vi "solar_voy Write (HS).vi"(4 "HDR_GUID":string, 6 "Suppress Errors? (T)":bool=TRUE, 7 "TARGET":string, 8 "error in (no error)":errorcluster, 10 "HANDSHAKE":T1, 11 "Voyager Refnum in":T2) -> (0 "error out":errorcluster, 3 "Voyager Refnum out":T2)   [LabVIEW 2018]
doc: "This writes the 'HANDSHAKE' packet used by the LINC interface."
uses:
  solar_voy_ctl Voyager Refnum.ctl
  solar_voy_def/solar_voy_def_ctl HANDSHAKE.ctl
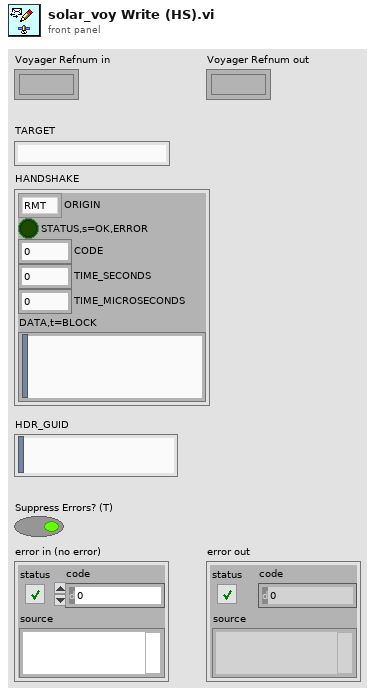
[diagram p1: front panel]
types:
  T1 = typedef "solar_voy_def_ctl HANDSHAKE.ctl" = cluster{"ORIGIN":enum8{"RMT", "LCL"}, "STATUS,s=OK,ERROR":bool, "CODE":i32, "TIME_SECONDS":u32, "TIME_MICROSECONDS":u32, "DATA,t=BLOCK":string}
  T2 = typedef "solar_voy_ctl Voyager Refnum.ctl" = refnum<k1>
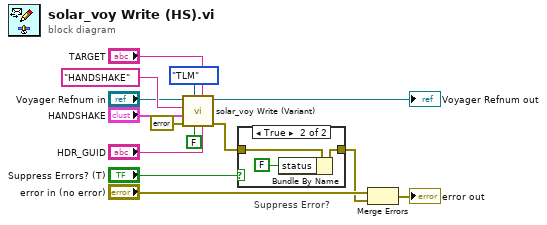
[diagram p0: block diagram]
diagram:
  n1 = call "solar_voy Write (Variant).vi"("HDR_GUID"="HDR_GUID", "TARGET"="TARGET", "Suppress Errors? (T)"=FALSE, "CMD"=enum8{"CMD", "TLM"}."TLM", "error in (no error)"=errorcluster {"status"=FALSE, "code"=0, "source"=""}, "Variant (No HDR)"="HANDSHAKE", "PACKET (\"\" = Use Variant)"="HANDSHAKE" ("PACKET (\"\" = Use Variant)"), "Voyager Refnum in"="Voyager Refnum in") -> ("error out"=w10:errorcluster, "Voyager Refnum out"=→"Voyager Refnum out":T2)  [unwired: 2 in]
  n2 = case "Suppress Error?" shown="True" "Suppress Errors? (T)" {
    tunnel: w10 -> [w15 w18]
    tunnel: [w15 w17] -> w12
    frame False {
    }
    frame True {
      n3 = Bundle By Name(cluster=w18, "status"=FALSE) -> (w17:errorcluster)
    }
  }
  n4 = Merge Errors("error in (no error)", w12) -> (→"error out":errorcluster)
